vi "Add MakerHub Feed.vi"(8 "Error In":errorcluster, 11 "Install LV Data":T1={"SSH Session"=refnum, "Status Log"="", "Detailed Log"="", "Credentials"={"Hostname or IP"="192.168.7.2", "Username"="root", "Password"=""}, "Target Info"={"OS Version"="", "CPU"="", "Systemd Version"="", "Internet Access"=FALSE, "Device Type"="", "LV Installed Ver"="", "LV Available Ver"="", "LV Upgrade Available"=FALSE, "Hostname"="", "NIC Info"=[]}, "Reboot Required?"=FALSE}) -> (0 "Error Out":errorcluster, 1 "Log":string, 3 "Install LV Data":T1={"SSH Session"=refnum, "Status Log"="", "Detailed Log"="", "Credentials"={"Hostname or IP"="192.168.7.2", "Username"="root", "Password"=""}, "Target Info"={"OS Version"="", "CPU"="", "Systemd Version"="", "Internet Access"=FALSE, "Device Type"="", "LV Installed Ver"="", "LV Available Ver"="", "LV Upgrade Available"=FALSE, "Hostname"="", "NIC Info"=[]}, "Reboot Required?"=FALSE})   [LabVIEW 2020, in "LMH-LINX.lvlib"]
uses:
  LMH-LINX.lvlib
  Install LV Data.ctl
  Target Info.ctl
  NIC Info.ctl
  NIC Mode.ctl
  <vilib>/regexp/Match Regular Expression.xnode
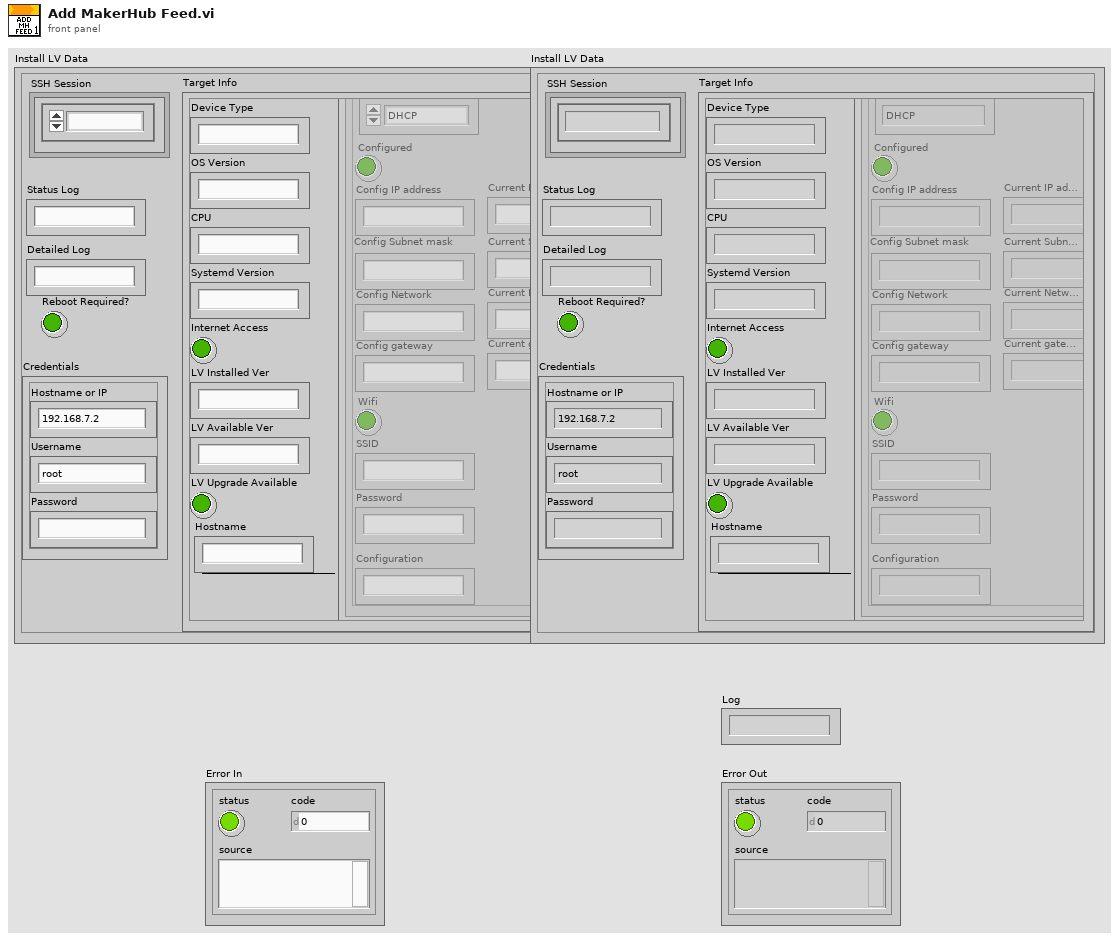
[diagram p1: front panel]
types:
  T1 = typedef "LMH-LINX.lvlib/Install LV Data.ctl" = cluster{"SSH Session":refnum<k1>, "Status Log":string, "Detailed Log":string, "Credentials":cluster{"Hostname or IP":string, "Username":string, "Password":string}, "Target Info":T2, "Reboot Required?":bool}
  T2 = typedef "LMH-LINX.lvlib/Target Info.ctl" = cluster{"OS Version":string, "CPU":string, "Systemd Version":string, "Internet Access":bool, "Device Type":string, "LV Installed Ver":string, "LV Available Ver":string, "LV Upgrade Available":bool, "Hostname":string, "NIC Info":T3[]}
  T3 = typedef "LMH-LINX.lvlib/NIC Info.ctl" = cluster{"Name":string, "NIC Mode":T4, "Configured":bool, "Config IP address":string, "Config Subnet mask":string, "Config Network":string, "Config gateway":string, "Wifi":bool, "SSID":string, "Password":string, "Configuration":string, "Current IP address":string, "Current Subnet mask":string, "Current gateway":string, "Current Network":string}
  T4 = typedef "LMH-LINX.lvlib/NIC Mode.ctl" = enum16{"DHCP", "Static", "Loopback"}
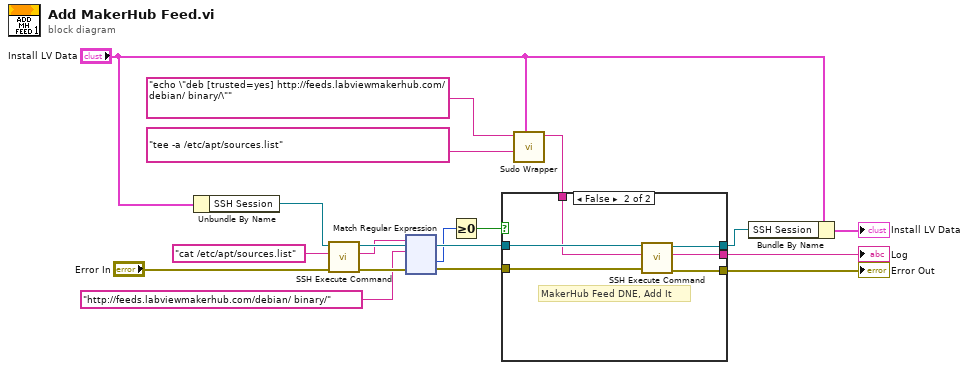
[diagram p0: block diagram]
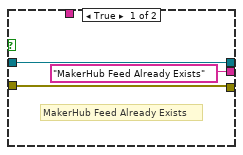
[diagram p2: hidden frame]
diagram:
  n1 = Unbundle By Name("Install LV Data") -> ("SSH Session"=w14:refnum<k1>)
  n2 = call "SSH Execute Command.vi"("Error In"="Error In", "Command"="cat /etc/apt/sources.list", "SSH Session"=w14) -> ("Error Out"=w9:errorcluster, "Std Out"=w10:string, "SSH Session"=w11:refnum<k1>)  [unwired: 6 in]
  n3 = xnode "Match Regular Expression"("input string"=w10, "regular expression"="http://feeds.labviewmakerhub.com/debian/ binary/", "error in"=w9) -> ("offset past match"=w6:i32, "error out"=w8:errorcluster)  [unwired: 3 in, 3 out]
  n4 = Greater Or Equal To 0?(x=w6) -> (x >= 0?=w5:bool)
  n5 = call "Sudo Wrapper.vi"("Install LV Data"="Install LV Data", "comand string"="tee -a /etc/apt/sources.list", "echo string"="echo \"deb [trusted=yes] http://feeds.labviewmakerhub.com/debian/ binary/\"") -> ("combined command string"=w2:string)  [unwired: 8 in]
  n6 = case shown="False" w5 {
    tunnel: ["MakerHub Feed Already Exists" ("Std Out") w27] -> w18
    tunnel: [w21 w26] -> w17
    tunnel: [w19 w25] -> w16
    tunnel: w11 -> [w19 w24]
    tunnel: w8 -> [w21 w23]
    tunnel: w2 -> [_ w22]
    frame True {
      # "MakerHub Feed Already Exists"
    }
    frame False {
      # "MakerHub Feed DNE, Add It"
      n7 = call "SSH Execute Command.vi"("Error In"=w23, "Command"=w22, "SSH Session"=w24) -> ("Error Out"=w26:errorcluster, "Std Out"=w27:string, "SSH Session"=w25:refnum<k1>)  [unwired: 6 in]
    }
  }
  "Log" <- w18
  "Error Out" <- w17
  n8 = Bundle By Name(cluster="Install LV Data", "SSH Session"=w16) -> (→"Install LV Data":T1)
